vi "ep_Power Correction.vi"   [LabVIEW 2024]
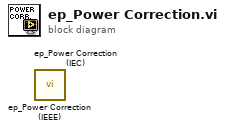
[diagram p0: block diagram]
diagram:
  n1 = call "ep_Power Correction (IEEE).vi"() -> ()  [unwired: 9 in, 3 out]
  n2 = call "ep_Power Correction (IEC).vi"() -> ()  [unwired: 9 in, 3 out]
